vi "PathPlanning.vi"(8 "Obstacle Map":dbl[][](array[numeric]), 11 "Target Point":cluster{"Target X":i32, "Target  Y":i32}) -> (3 "Planned Path":T1)   [LabVIEW 2011]
uses:
  <vilib>/robotics/Navigation/shared/WorldMap/OccupancyGridWorldMap/NI_Robotics_OccupancyGridWorldMap.lvclass
  <vilib>/robotics/Navigation/NI_Robotics_Navigation .lvlib
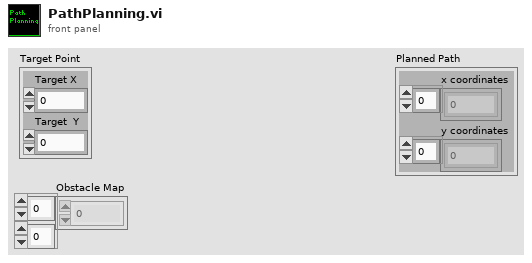
[diagram p1: front panel]
types:
  T1 = cluster{"x coordinates":i32[], "y coordinates":i32[]}
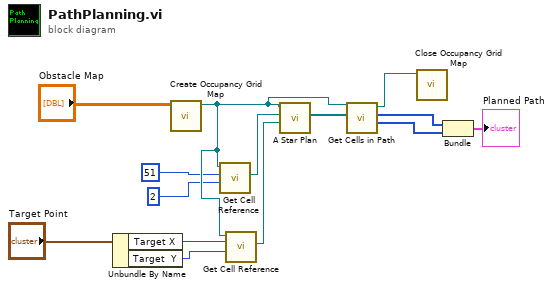
[diagram p0: block diagram]
diagram:
  n1 = Unbundle By Name("Target Point") -> ("Target X"=w6:i32, "Target  Y"=w7:i32)
  n2 = call <vilib>:"Create Occupancy Grid Map.vi"("occupancy grid"="Obstacle Map") -> ("map reference out"=w11:refnum<data-value>)  [unwired: 9 in, 1 out]
  n3 = call <vilib>:"Get Cell Reference.vi"("y"=2, "x"=51, "map reference in"=w11) -> ("cell reference"=w14:refnum<data-value>)  [unwired: 5 in, 3 out]
  n4 = call <vilib>:"Get Cell Reference.vi"("y"=w7, "x"=w6, "map reference in"=w11) -> ("cell reference"=w13:refnum<data-value>)  [unwired: 5 in, 3 out]
  n5 = call <vilib>:"A Star Plan.vi"("goal reference"=w13, "start reference"=w14, "map reference in"=w11) -> ("path references"=w12:refnum<data-value>[])  [unwired: 5 in, 3 out]
  n6 = call <vilib>:"Get Cells in Path.vi"("path references"=w12, "map reference in"=w11) -> ("y coordinates"=w2:i32[], "x coordinates"=w3:i32[], "map reference out"=w8:refnum<data-value>)  [unwired: 6 in, 1 out]
  n7 = call <vilib>:"Close Occupancy Grid Map.vi"("map reference in"=w8) -> ()  [unwired: 10 in, 1 out]
  n8 = Bundle("x coordinates"=w3, "y coordinates"=w2) -> (→"Planned Path":T1)  [unwired: 1 in]
